vi "Read Depth Tiny Resolution.vi"(8 "error in (no error)":errorcluster) -> (0 "error out":errorcluster, 3 "Depth image":picture)   [LabVIEW 2017]
uses:
  libkinect_wrapper.dll
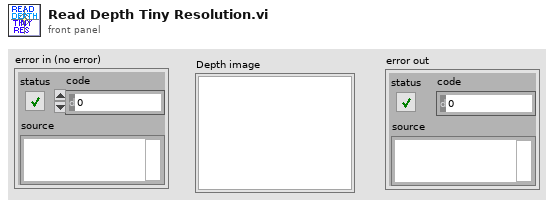
[diagram p1: front panel]
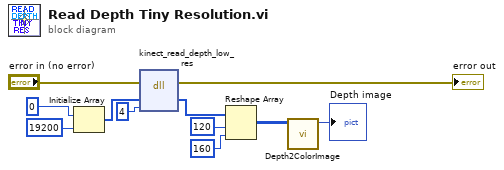
[diagram p0: block diagram]
diagram:
  n1 = Initialize Array(u16 0 ("element"), 19200) -> (w11:u16[])
  n2 = dll-call lib="libkinect_wrapper.*" fn="kinect_read_depth_low_res"(error in="error in (no error)", "depth"=w11, "factor"=4) -> (error out=→"error out":errorcluster, "depth"=w6:u16[])  [unwired: 4 in, 1 out]
  n3 = Reshape Array(w6, 120 ("dimension size"), 160 ("dimension size")) -> (w2:u16[][])
  n4 = call "Depth2ColorImage.vi"("Depth"=w2) -> ("HSV Image"=→"Depth image":picture)  [unwired: 10 in]
